vi "Activate Panel VI.vi"(8 "error in (no error)":errorcluster, 11 "Console in":refnum<class "Console.lvclass">) -> (0 "error out":errorcluster, 3 "Console out":refnum<class "Console.lvclass">)   [LabVIEW 2015, in "EditPanel API.lvlib" / "Console.lvclass"]
uses:
  Console.lvclass
  Console.lvclass/Console.ctl
  Console Reply/Console Reply/Console Reply.lvclass/Console Reply.ctl
  Console Reply/Console Reply/Console Reply.lvclass
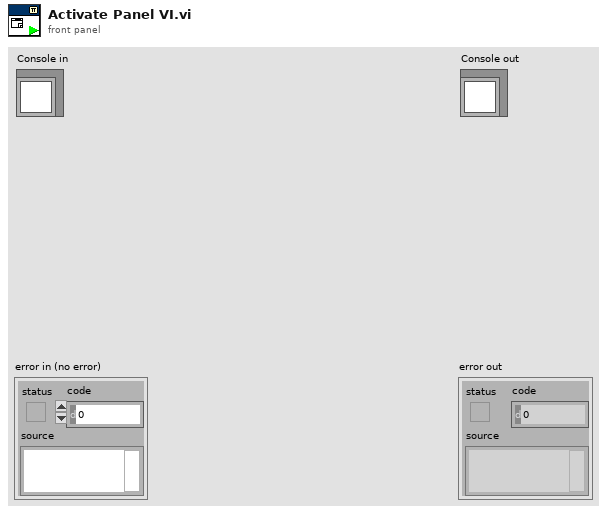
[diagram p1: front panel]
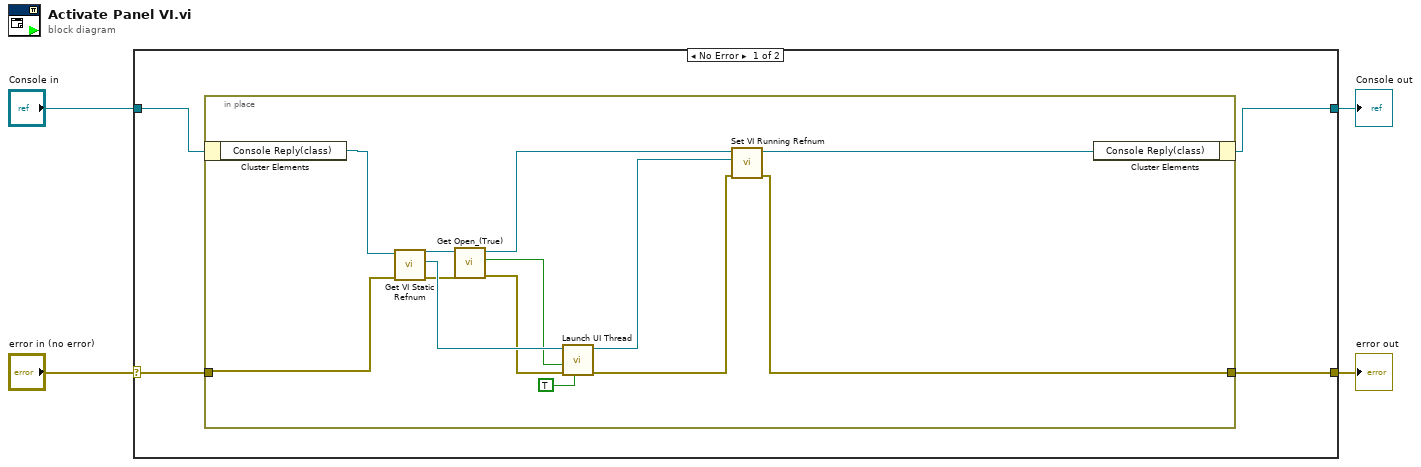
[diagram p0: block diagram]
diagram:
  n1 = case shown="No Error" "error in (no error)" {
    selector: "error in (no error)" -> [w8 w23]
    tunnel: [w5 w23] -> w3
    tunnel: [w7 w22] -> w1
    tunnel: "Console in" -> [w6 w22]
    frame No Error {
      n2 = in-place {
        in-place-border: w8 -> [w16]
        in-place-border: [w18] -> w5
        n3 = in-place-cluster #1(w6) -> ("Console Reply(class)"=w17:refnum<class "Console Reply.lvclass">)
        n4 = call "Get VI Static Refnum.vi"("error in (no error)"=w16, "Console Reply in"=w17) -> ("error out"=w13:errorcluster, "VI Static Refnum"=w15:refnum<vi>, "Console Reply out"=w14:refnum<class "Console Reply.lvclass">)  [unwired: 7 in]
        n5 = call "Get Open_(True).vi"("error in (no error)"=w13, "Console Reply in"=w14) -> ("error out"=w11:errorcluster, "Open?(True)"=w12:bool, "Console Reply out"=w10:refnum<class "Console Reply.lvclass">)  [unwired: 7 in]
        n6 = call "Launch UI Thread.vi"("SubPanel?(False)"=TRUE, "error in (no error)"=w11, "Open?(True)"=w12, "This VI"=w15) -> ("error out"=w20:errorcluster, "VI Running Refnum"=w21:refnum<vi>)  [unwired: 6 in]
        n7 = call "Set VI Running Refnum.vi"("error in (no error)"=w20, "VI Running Refnum"=w21, "Console Reply.lvclass"=w10) -> ("error out"=w18:errorcluster, "Console Reply.lvclass out"=w19:refnum<class "Console Reply.lvclass">)  [unwired: 7 in]
        n8 = in-place-cluster #1("Console Reply(class)"=w19) -> (w7:refnum<class "Console.lvclass">)
      }
    }
    frame Error {
    }
  }
  "error out" <- w3
  "Console out" <- w1
